vi "Format SQL INSERT.vi"(6 "Time Stamp":timestamp, 8 "error in":errorcluster, 9 "Data":variant, 10 "Path(s)":variant, 11 "LV-Data.PGSQL in":refnum<class "LV-Data.PGSQL.lvclass">) -> (0 "error out":errorcluster, 1 "Paths out":string, 2 "Formatted Insert":string, 3 "LV-Data.PGSQL out":refnum<class "LV-Data.PGSQL.lvclass">)   [LabVIEW 2019, in "LV-Data.PGSQL.lvclass"]
uses:
  LV-Data.PGSQL.lvclass
  <vilib>/ErrorRing/Error Ring.xnode
  <vilib>/Utility/error.llb/Error Cluster From Error Code.vi
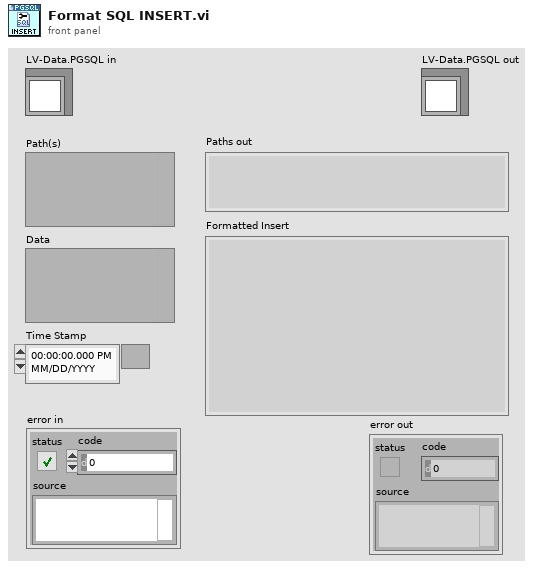
[diagram p1: front panel]
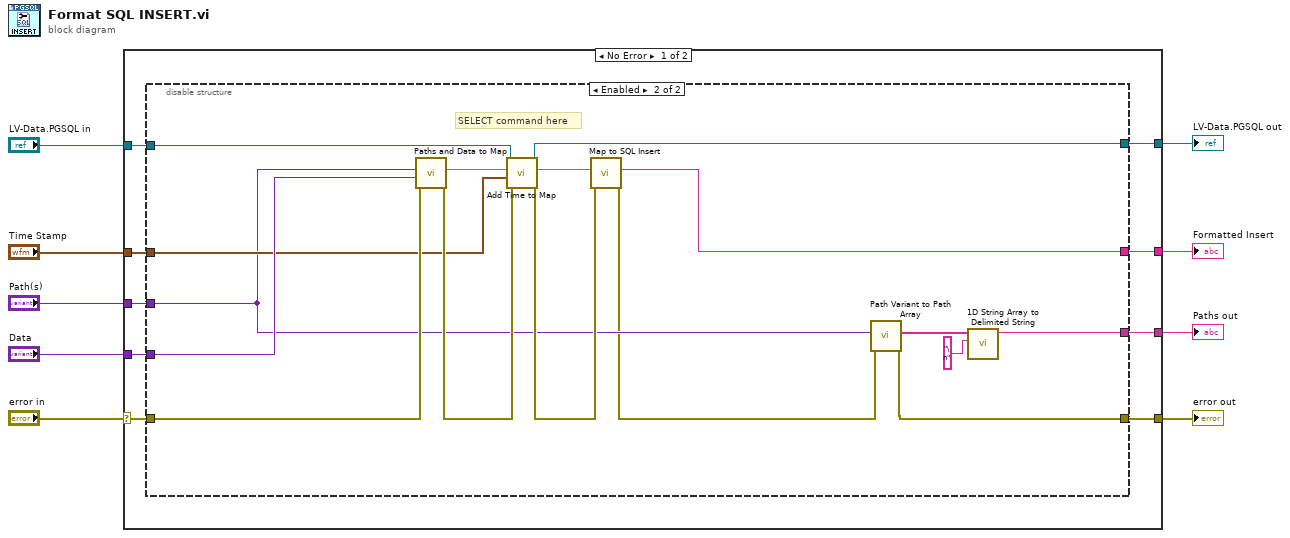
[diagram p0: block diagram]
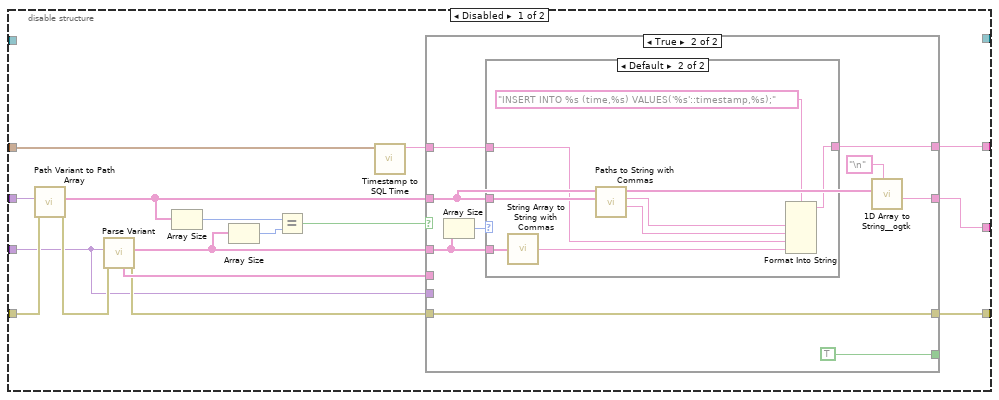
[diagram p2: hidden frame]
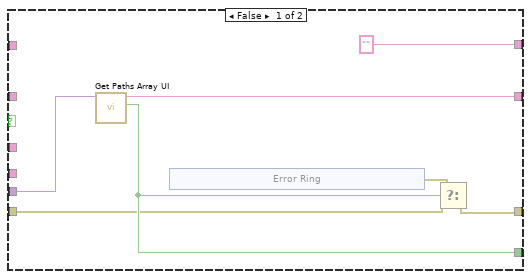
[diagram p3: hidden frame]
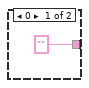
[diagram p4: hidden frame]
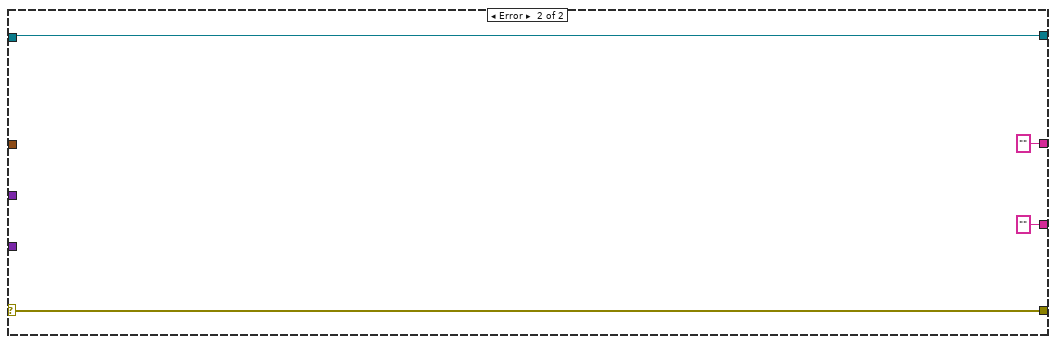
[diagram p5: hidden frame]
diagram:
  n1 = case shown="No Error" "error in" {
    selector: "error in" -> [w15 w84]
    tunnel: [w18 w84] -> w9
    tunnel: "Path(s)" -> [w17 _]
    tunnel: [w16 "" ("delimited string")] -> w7
    tunnel: "Time Stamp" -> [w14 _]
    tunnel: "Data" -> [w13 _]
    tunnel: [w12 "" ("delimited string")] -> w3
    tunnel: "LV-Data.PGSQL in" -> [w11 w83]
    tunnel: [w10 w83] -> w1
    frame No Error {
      n2 = disable-structure shown="Enabled" {
        disable-tunnel: w17 -> [w33 w70]
        disable-tunnel: [w32 w72] -> w16
        disable-tunnel: w14 -> [w25 w73]
        disable-tunnel: w13 -> [w21 w74]
        disable-tunnel: [w19 w66] -> w12
        disable-tunnel: w11 -> [_ w79]
        disable-tunnel: [_ w78] -> w10
        disable-tunnel: w15 -> [w31 w77]
        disable-tunnel: [w34 w68] -> w18
        frame Disabled {
          n3 = call "Path Variant to Path Array.vi"("error in"=w31, "Paths"=w33) -> ("error out"=w30:errorcluster, "Paths"=w26:string[])  [unwired: 8 in]
          n4 = call "Parse Variant.vi"("error in"=w30, "Data"=w21) -> ("error out"=w27:errorcluster, "Data"=w22:string[], "Type (Name)"=w28:string[])  [unwired: 5 in, 2 out]
          n5 = Array Size(array=w26) -> (size(s)=w24:i32)
          n6 = Array Size(array=w22) -> (size(s)=w23:i32)
          n7 = Equal?(x=w24, y=w23) -> (x = y?=w35:bool)
          n8 = call "Timestamp to SQL Time.vi"("Timestamp"=w25) -> ("date/time string"=w29:string)  [unwired: 10 in]
          n9 = case shown="True" w35 {
            tunnel: w26 -> [_ w48]
            tunnel: [w37 w55] -> w34
            tunnel: w27 -> [w36 w55]
            tunnel: w29 -> [_ w54]
            tunnel: w28 -> [_ _]
            tunnel: ["" w50] -> w32
            tunnel: w22 -> [_ w53]
            tunnel: w21 -> [w41 _]
            tunnel: [w38 TRUE] -> w20
            tunnel: [w40 w47] -> w19
            frame False {
              n10 = call "Get Paths Array UI.vi"("Data"=w41) -> ("Cancelled?"=w38:bool, "selected_paths"=w40:string)  [unwired: 9 in]
              n11 = xnode "Error Ring"() -> ("error out"=w39:errorcluster)
              n12 = Select(t=w39, s=w38, f=w36) -> (s? t:f=w37:errorcluster)
            }
            frame True {
              n13 = Array Size(array=w53) -> (size(s)=w52:i32)
              n14 = case shown="Default" w52 {
                tunnel: w48 -> [_ w64]
                tunnel: ["" w60] -> w50
                tunnel: w54 -> [_ w58]
                tunnel: w53 -> [_ w57]
                frame 0 {
                }
                frame Default {
                  n15 = call "String Array to String with Commas.vi"("Array"=w57) -> ("String"=w61:string)
                  n16 = call "Paths to String with Commas.vi"("Paths"=w64) -> ("Columns"=w62:string, "Table"=w63:string)  [unwired: 9 in]
                  n17 = Format Into String(format string="INSERT INTO %s (time,%s) VALUES('%s'::timestamp,%s);", w63, w62, w58, w61) -> (resulting string=w60:string)  [unwired: 2 in, 1 out]
                }
              }
              n18 = call <userlib>:"1D Array to String__ogtk.vi"("delimiter (Tab)"="\n", "Array of Strings"=w48) -> ("delimited string"=w47:string)  [unwired: 9 in]
            }
          }
        }
        frame Enabled {
          # "SELECT command here"
          n19 = call "Paths and Data to Map.vi"("error in"=w77, "Data"=w74, "Paths"=w70) -> ("error out"=w76:errorcluster, "map out"=w80:map{string, map{string, string[]}})  [unwired: 6 in, 1 out]
          n20 = call "Add Time to Map.vi"("error in (no error)"=w76, "Times"=w73, "map in"=w80, "LV-Data.PGSQL in"=w79) -> ("error out"=w75:errorcluster, "map out"=w71:map{string, map{string, string[]}}, "LV-Data.PGSQL out"=w78:refnum<class "LV-Data.PGSQL.lvclass">)  [unwired: 5 in]
          n21 = call "Map to SQL Insert.vi"("error in (no error)"=w75, "map in"=w71) -> ("error out"=w69:errorcluster, "delimited string"=w72:string)  [unwired: 8 in]
          n22 = call "Path Variant to Path Array.vi"("error in"=w69, "Paths"=w70) -> ("error out"=w68:errorcluster, "Paths"=w67:string[])  [unwired: 8 in]
          n23 = call <vilib>:"1D String Array to Delimited String.vi"("delimiter"="\n", "string array"=w67) -> ("delimited string"=w66:string)  [unwired: 9 in]
        }
      }
    }
    frame Error {
    }
  }
  "error out" <- w9
  "Formatted Insert" <- w7
  "Paths out" <- w3
  "LV-Data.PGSQL out" <- w1
